vi "Print raw data to url.vi"(8 "error in":errorcluster, 10 "ZPL text to print":string, 11 "Printer name url":string) -> (0 "error out":errorcluster, 3 "Print Label OK?":bool=TRUE)   [LabVIEW 2013]
panel:
  out "IP":string
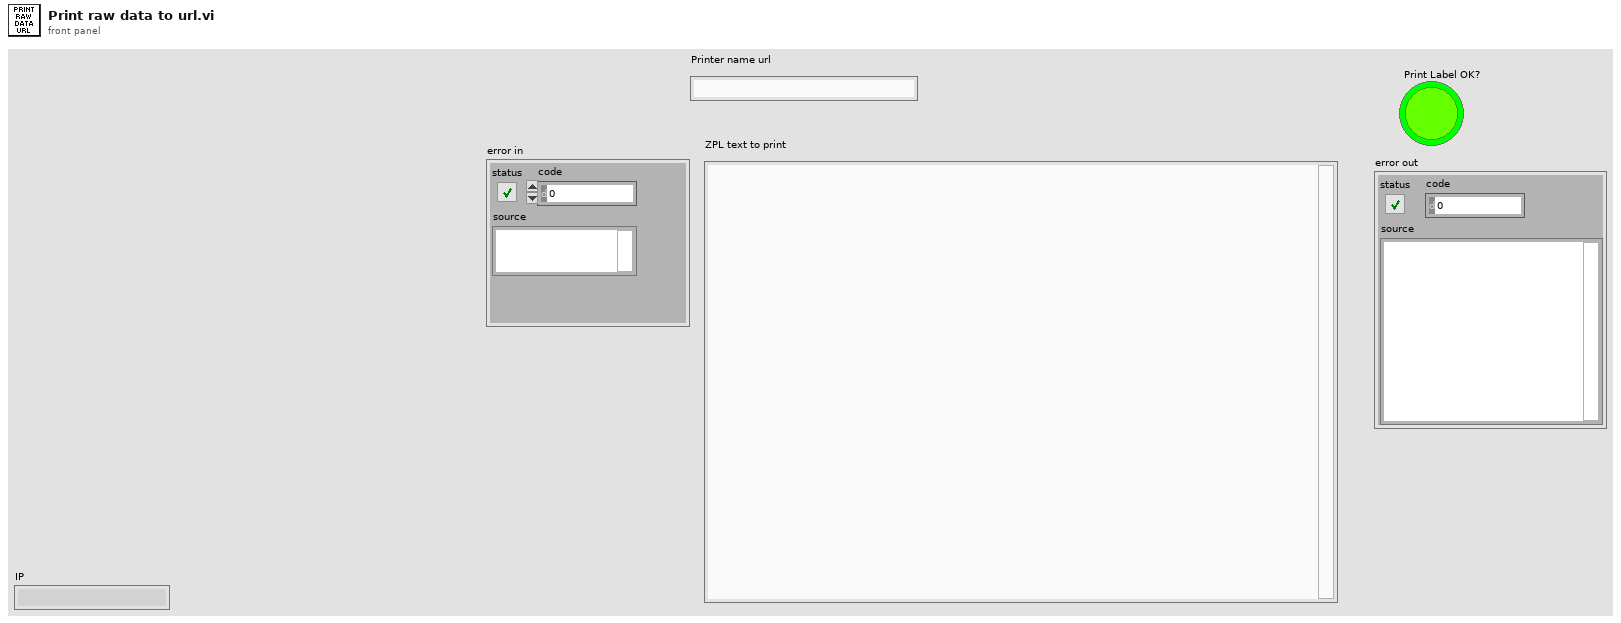
[diagram p1: front panel]
types:
  T1 = cluster{"Test folder":string, "Top level":string, "Main":string, "Test report":string, "Work order qty":string, "Work order meid":string, "Work order imei":string, "Master meid imei list":string, "Master test data":string, "ZPL label info":string, "Pictures":string, "Setup info":string, "Work order":string, "Tests folder":string, "Tests steps folder":string, "Config folder":string, "Verizon Upload file":string, "Job data file":string, "Station globals":string, "Post test info":string}
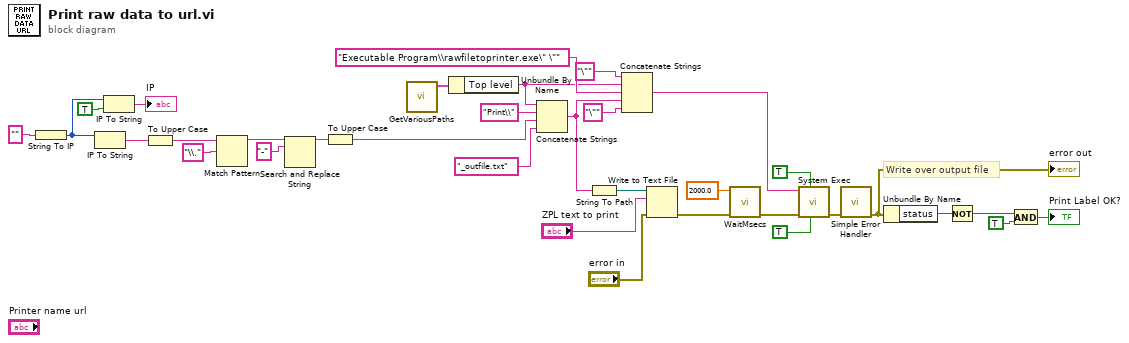
[diagram p0: block diagram]
diagram:
  # "Write over output file"
  n1 = String To IP(1:"" ("name")) -> (0:w16:u32)
  n2 = IP To String(2:w16) -> (0:w10:string)  [unwired: 1 in]
  n3 = IP To String(1:TRUE ("dot notation? (F)"), 2:w16) -> (0:→"IP":string)
  n4 = To Upper Case(1:w10) -> (0:w9:string)
  n5 = Match Pattern(string=w9, regular expression="\\.") -> (before substring=w13:string)  [unwired: 1 in, 3 out]
  n6 = Search and Replace String(input string=w13, search string="-") -> (result string=w11:string)  [unwired: 6 in, 3 out]
  n7 = To Upper Case(1:w11) -> (0:w8:string)
  n8 = call "GetVariousPaths.vi"() -> ("Built Paths"=w29:T1)  [unwired: 10 in, 1 out]
  n9 = Unbundle By Name(w29) -> ("Top level"=w26:string)
  n10 = Concatenate Strings(w26, "Print\\" ("string"), w8, "_outfile.txt" ("string")) -> (w20:string)
  n11 = String To Path(string=w20) -> (path=w5:path)
  n12 = Concatenate Strings("\"" ("string"), w26, "Executable Program\\rawfiletoprinter.exe\" \"" ("string"), w20, "\"" ("string")) -> (w1:string)
  n13 = Write to Text File(file (use dialog)=w5, text="ZPL text to print", error in="error in") -> (error out=w2:errorcluster)  [unwired: 1 in, 2 out]
  n14 = call "WaitMsecs.vi"("error in (no error)"=w2, "Wait Msecs"=2000.0) -> ("error out"=w7:errorcluster)  [unwired: 9 in]
  n15 = call <vilib>:"System Exec.vi"("run minimized? (F)"=TRUE, "wait until completion? (T)"=TRUE, "error in (no error)"=w7, "command line"=w1) -> ("error out"=w19:errorcluster)  [unwired: 4 in, 3 out]
  n16 = call <vilib>:"Simple Error Handler.vi"("error in (no error)"=w19) -> ("error out"=w24:errorcluster)  [unwired: 4 in, 4 out]
  "error out" <- w24
  n17 = Unbundle By Name(w24) -> ("status"=w32:bool)
  n18 = Not(x=w32) -> (.not. x?=w31:bool)
  n19 = And(x=w31, y=TRUE) -> (x .and. y?=→"Print Label OK?":bool)
